vi "Grove RGB I2C LCD Full.vi"() -> ()   [LabVIEW 2020, in "CTI-Scratchpad.lvlib"]
uses:
  CTI-Scratchpad.lvlib
  CTI-Peripheral/Character LCD/Position.ctl
  CTI-Peripheral/Character LCD/Custom Char.ctl
  CTI/Identity.ctl
  CTI/GPIO Number.ctl
  CTI/I2C Number.ctl
  CTI-Peripheral/Grove I2C LCD/Grove I2C LCD.lvclass
  C:/Users/Public/Github/cti-drivers-lv-visa/CTI-Peripheral/Character LCD/Char LCD.lvclass
  CTI-Peripheral/RGB I2C/Grove I2C RGB SGM31323/Grove I2C RGB SGM31323.lvclass
  CTI/Session/Session.lvclass
  CTI/VisaComms/VisaComms.lvclass
  CTI-Peripheral/Character LCD/Char LCD.lvclass
  CTI/CTI.lvlib
panel:
  in  "SetBacklight":bool
  in  "Grove Connector":enum16{"I2C0", "I2C1"}(ring)
  in  "RGBBacklight":u32(colorbox)=16775281
  out "Identity":T1
  in  "Custom Chars":T3
  in  "Create":bool
  in  "stop":bool
  out "error out":errorcluster
  in  "Scroll Right":bool
  in  "Scroll Left":bool
  in  "Home":bool
  in  "Clear":bool
  in  "Write Text":bool
  in  "Text":string="Hello LabVIEW!"
  in  "Port":refnum<visa-resource-name>="COM5"
  in  "Goto":bool
  in  "Position":T4
  in  "Display":bool=TRUE
  in  "Blink":bool
  in  "Cursor":bool=TRUE
  # "Use \\00 through \\07 to specify custom chars"
  # "https://www.seeedstudio.com/Grove-LCD-RGB-Backlight.html"
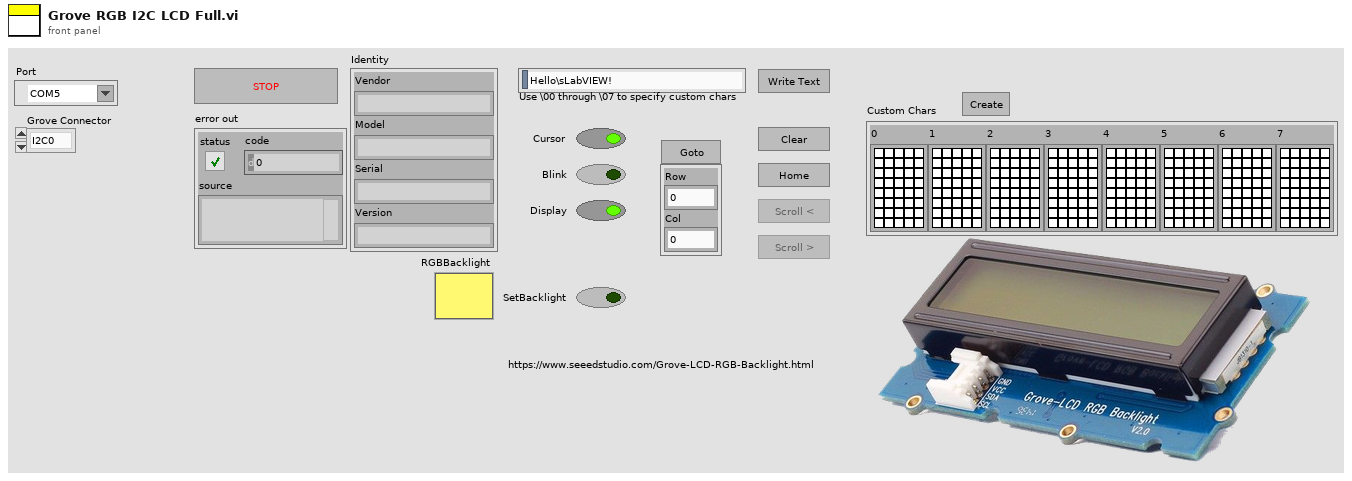
[diagram p1: front panel]
types:
  T1 = typedef "CTI.lvlib/Identity.ctl" = cluster{"Vendor":string, "Model":string, "Serial":string, "Version":string}
  T2 = typedef "CTI-Peripheral.lvlib/Char LCD.lvclass/Custom Char.ctl" = bool[][]
  T3 = cluster{"0":T2, "1":T2, "2":T2, "3":T2, "4":T2, "5":T2, "6":T2, "7":T2}
  T4 = typedef "CTI-Peripheral.lvlib/Char LCD.lvclass/Position.ctl" = cluster{"Row":u8, "Col":u8}
  T5 = typedef "CTI.lvlib/I2C Number.ctl" = i8
  T6 = typedef "CTI.lvlib/GPIO Number.ctl" = i8
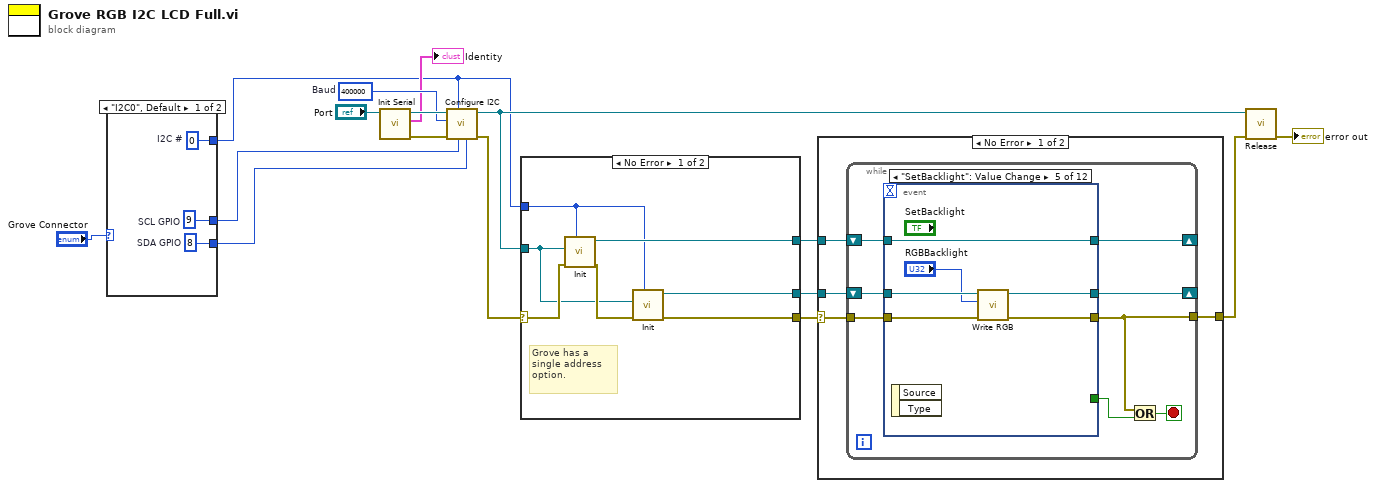
[diagram p0: block diagram]
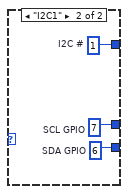
[diagram p2: hidden frame]
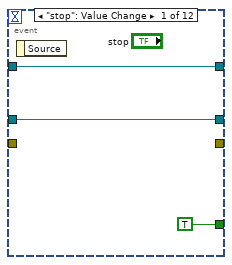
[diagram p4: hidden frame]
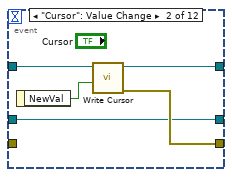
[diagram p5: hidden frame]
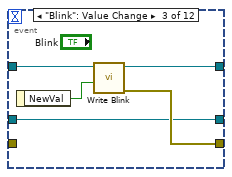
[diagram p6: hidden frame]
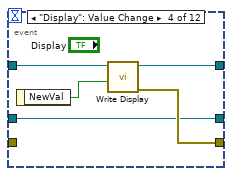
[diagram p7: hidden frame]
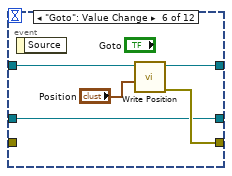
[diagram p8: hidden frame]
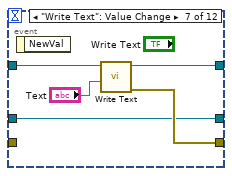
[diagram p9: hidden frame]
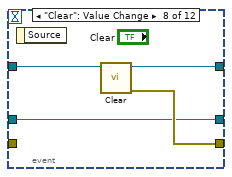
[diagram p10: hidden frame]
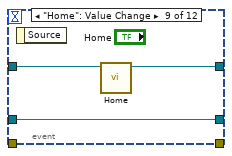
[diagram p11: hidden frame]
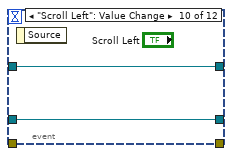
[diagram p12: hidden frame]
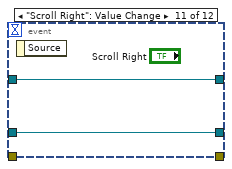
[diagram p13: hidden frame]
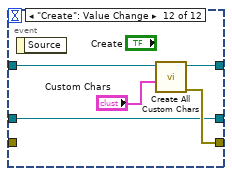
[diagram p14: hidden frame]
diagram:
  w8 = u32 400000  # Baud
  n1 = case shown="\"I2C0\", Default" "Grove Connector" {
    tunnel: [w19 w22] -> w3
    tunnel: [w18 w21] -> w2
    tunnel: [w17 w20] -> w4
    frame "I2C0", Default {
      w17 = T5 0  # I2C #
      w18 = T6 8  # SDA GPIO
      w19 = T6 9  # SCL GPIO
    }
    frame "I2C1" {
      w20 = T5 1  # I2C #
      w21 = T6 6  # SDA GPIO
      w22 = T6 7  # SCL GPIO
    }
  }
  n2 = call "Init Serial.vi"("VISA resource name in"="Port") -> ("error out"=w15:errorcluster, "Identity"=→"Identity":T1, "Session"=w9:refnum<class "Session.lvclass">)  [unwired: 8 in]
  n3 = call "Configure I2C.vi"("SDA GPIO"=w2, "SCL GPIO"=w3, "I2C #"=w4, "error in (no error)"=w15, "Baud"=w8, "Session in"=w9) -> ("error out"=w10:errorcluster, "Session out"=w6:refnum<class "Session.lvclass">)  [unwired: 4 in]
  n4 = case shown="No Error" w10 {
    selector: w10 -> [w28 w30]
    tunnel: [w24 w30] -> w14
    tunnel: [w29 _] -> w13
    tunnel: w6 -> [w26 _]
    tunnel: w4 -> [w25 _]
    tunnel: [w23 _] -> w1
    frame No Error {
      # "Grove has a single address option."
      n5 = call "Init.vi"("I2C #"=w25, "error in (no error)"=w28, "Session In"=w26) -> ("error out"=w27:errorcluster, "Grove I2C LCD out"=w29:refnum<class "Grove I2C LCD.lvclass">)  [unwired: 7 in]
      n6 = call "Init.vi"("I2C #"=w25, "error in (no error)"=w27, "Session In"=w26) -> ("error out"=w24:errorcluster, "Grove I2C RGB SGM31323 Out"=w23:refnum<class "Grove I2C RGB SGM31323.lvclass">)  [unwired: 7 in]
    }
    frame Error {
    }
  }
  n7 = case shown="No Error" w14 {
    selector: w14 -> [w31 w93]
    tunnel: w13 -> [w34 _]
    tunnel: [w33 w93] -> w12
    tunnel: w1 -> [w32 _]
    frame No Error {
      n8 = while {
        shift-right: [w38] -> _
        shift-left: w34 -> [w42]
        tunnel: [w39] -> w33
        shift-right: [w36] -> _
        shift-left: w32 -> [w37]
        tunnel: w31 -> [w35]
        stop <- w40 stop-if-true
        n9 = event shown="[4] \"SetBacklight\": Value Change" {
          selector: _ -> [_ _ _ _ _ _ _ _ _ _ _ _]
          dyn-events: _ -> [_ _ _ _ _ _ _ _ _ _ _ _]
          timeout: _ -> [_ _ _ _ _ _ _ _ _ _ _ _]
          tunnel: w42 -> [w45 w47 w52 w57 w66 w68 w73 w78 w82 w85 w87 w89]
          tunnel: [w45 w50 w55 w60 w66 w69 w75 w80 w83 w85 w87 w92] -> w38
          tunnel: [TRUE _ _ _ _ _ _ _ _ _ _ _] -> w41
          tunnel: [_ w48 w53 w58 w62 w70 w74 w79 _ _ _ w91] -> w39
          tunnel: w37 -> [w43 w46 w51 w56 w64 w67 w72 w77 w81 w84 w86 w88]
          tunnel: [w43 w46 w51 w56 w63 w67 w72 w77 w81 w84 w86 w88] -> w36
          tunnel: w35 -> [_ _ _ _ w65 _ _ _ _ _ _ _]
          event "stop": Value Change {
            n10 = event-data() -> ()  [unwired: 1 in, 1 out]
          }
          event "Cursor": Value Change {
            n11 = event-data() -> ("NewVal"=w49:bool)  [unwired: 1 in]
            n12 = call-dynamic "Write Cursor.vi"("Cursor On"=w49, "Grove I2C LCD I in"=w47) -> ("error out"=w48:errorcluster, "Grove I2C LCD I out"=w50:refnum<class "Grove I2C LCD.lvclass">)  [unwired: 8 in]
          }
          event "Blink": Value Change {
            n13 = event-data() -> ("NewVal"=w54:bool)  [unwired: 1 in]
            n14 = call-dynamic "Write Blink.vi"("Blink On"=w54, "Grove I2C LCD I in"=w52) -> ("error out"=w53:errorcluster, "Grove I2C LCD I out"=w55:refnum<class "Grove I2C LCD.lvclass">)  [unwired: 8 in]
          }
          event "Display": Value Change {
            n15 = event-data() -> ("NewVal"=w59:bool)  [unwired: 1 in]
            n16 = call-dynamic "Write Display.vi"("Display On"=w59, "Grove I2C LCD I in"=w57) -> ("error out"=w58:errorcluster, "Grove I2C LCD I out"=w60:refnum<class "Grove I2C LCD.lvclass">)  [unwired: 8 in]
          }
          event "SetBacklight": Value Change {
            n17 = event-data() -> ()  [unwired: 1 in, 2 out]
            n18 = call-dynamic "Write RGB.vi"("error in (no error)"=w65, "Color Box"="RGBBacklight", "Grove I2C RGB SGM31323 in"=w64) -> ("error out"=w62:errorcluster, "Grove I2C RGB SGM31323 out"=w63:refnum<class "Grove I2C RGB SGM31323.lvclass">)  [unwired: 7 in]
          }
          event "Goto": Value Change {
            n19 = event-data() -> ()  [unwired: 1 in, 1 out]
            n20 = call-dynamic "Write Position.vi"("Position"="Position", "Grove I2C LCD I in"=w68) -> ("error out"=w70:errorcluster, "Grove I2C LCD I out"=w69:refnum<class "Grove I2C LCD.lvclass">)  [unwired: 8 in]
          }
          event "Write Text": Value Change {
            n21 = event-data() -> ()  [unwired: 1 in, 1 out]
            n22 = call-dynamic "Write Text.vi"("Text"="Text", "Character LCD in"=w73) -> ("error out"=w74:errorcluster, "Character LCD out"=w75:refnum<class "Grove I2C LCD.lvclass">)  [unwired: 8 in]
          }
          event "Clear": Value Change {
            n23 = event-data() -> ()  [unwired: 1 in, 1 out]
            n24 = call-dynamic "Clear.vi"("Character LCD in"=w78) -> ("error out"=w79:errorcluster, "Character LCD out"=w80:refnum<class "Grove I2C LCD.lvclass">)  [unwired: 9 in]
          }
          event "Home": Value Change {
            n25 = event-data() -> ()  [unwired: 1 in, 1 out]
            n26 = call-dynamic "Home.vi"("Character LCD in"=w82) -> ("Character LCD out"=w83:refnum<class "Grove I2C LCD.lvclass">)  [unwired: 9 in, 1 out]
          }
          event "Scroll Left": Value Change {
            n27 = event-data() -> ()  [unwired: 1 in, 1 out]
          }
          event "Scroll Right": Value Change {
            n28 = event-data() -> ()  [unwired: 1 in, 1 out]
          }
          event "Create": Value Change {
            n29 = event-data() -> ()  [unwired: 1 in, 1 out]
            n30 = call "Create All Custom Chars.vi"("Custom Chars"="Custom Chars", "Char LCD in"=w89) -> ("error out"=w91:errorcluster, "Char LCD out"=w92:refnum<class "Grove I2C LCD.lvclass">)  [unwired: 8 in]
          }
        }
        n31 = Or(x=w39, y=w41) -> (x .or. y?=w40:bool)
      }
    }
    frame Error {
    }
  }
  n32 = call-dynamic "Release.vi"("error in (no error)"=w12, "Session in"=w6) -> ("error out"=→"error out":errorcluster)  [unwired: 9 in]
